vi "String_Write Index.vi"(9 "Value":string, 11 "Index":i32) -> ()   [LabVIEW 2010, in "Current Value Table.lvlib"]
doc: "This VI takes a memory index (I32) and will perform a write on that index. This VI has no error handling for increased performance. If the index is invalid, no data will be transferred."
uses:
  Current Value Table.lvlib
  Type Defs/Memory Commands.ctl
  String_Memory Block.vi
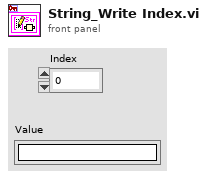
[diagram p1: front panel]
types:
  T1 = typedef "Current Value Table.lvlib/Memory Commands.ctl" = enum16{"Init", "Add Data", "Read", "Read Group", "Read All", "Write", "Write Group", "Get Size"}
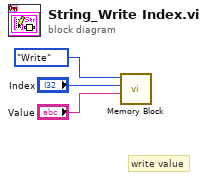
[diagram p0: block diagram]
diagram:
  # "write value"
  n1 = call-poly "Memory Block.vi"("Value"="Value", "Index"="Index", "Method"=Memory_Commands."Write") -> ()  [unwired: 6 in, 3 out]
